vi "Status Alarms.vi"(8 "error in":errorcluster, 11 "Network Path In":string="192.168.169.1") -> (0 "error out":errorcluster, 2 "Data":i16[](array[numeric]), 3 "Network Path Out":string="192.168.169.1")   [LabVIEW 2018]
doc: "Lee toda la tabla de memoria Status.Alarms del equipo PowerMonitor 5000."
uses:
  <vilib>/ethernetip/ethernetip.llb/EthernetIP SLC500 Read Integer.vi
  <vilib>/ethernetip/ethernetip.lvlib
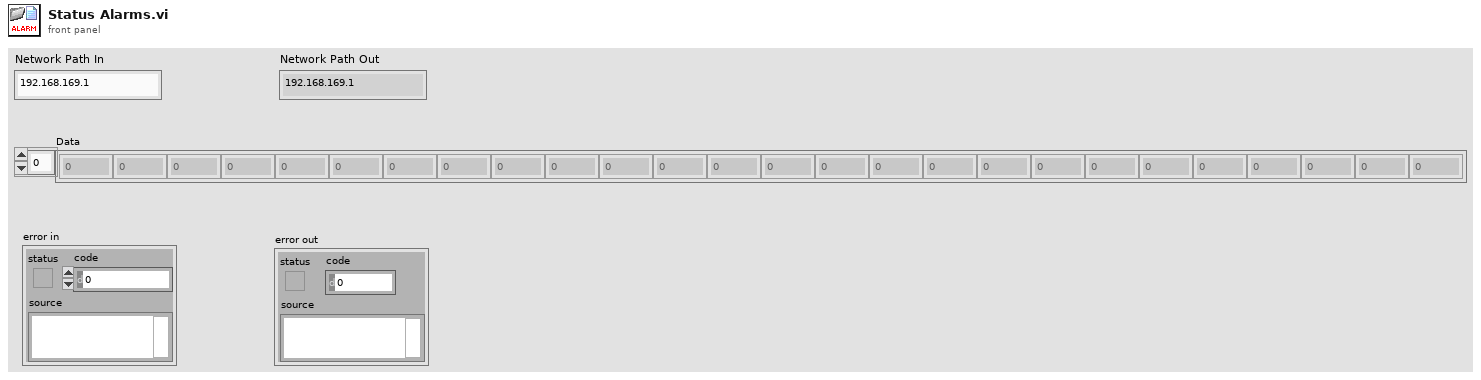
[diagram p1: front panel]
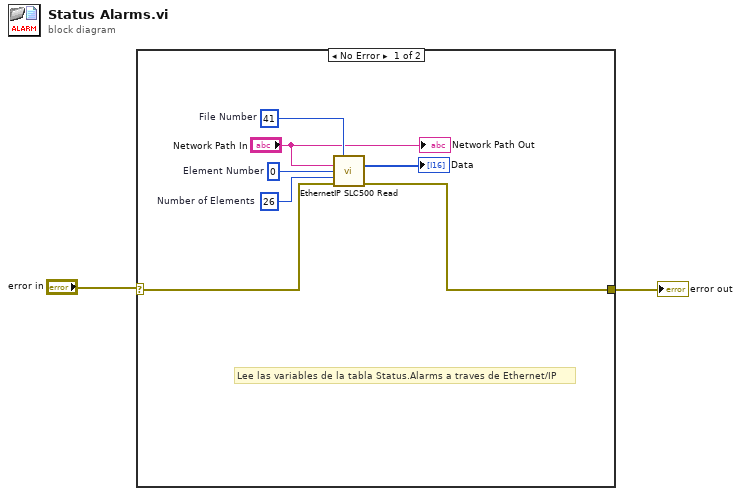
[diagram p0: block diagram]
diagram:
  n1 = case shown="No Error" "error in" {
    selector: "error in" -> [w3 w10]
    tunnel: [w6 w10] -> w2
    frame No Error {
      w7 = u32 26  # Number of Elements
      w9 = u16 41  # File Number
      w8 = u16 0  # Element Number
      # "Lee las variables de la tabla Status.Alarms a traves de Ethernet/IP"
      n2 = call-poly <vilib>:"EthernetIP SLC500 Read.vi"("File Number"=w9, "Network Path"="Network Path In", "Element Number"=w8, "Number of Elements"=w7, "error in"=w3) -> ("Data"=→"Data":i16[], "error out"=w6:errorcluster)  [unwired: 8 in, 1 out]
      "Network Path Out" <- "Network Path In"
    }
    frame Error {
    }
  }
  "error out" <- w2
